vi "Router - Latency Bmk - Queue.vi"() -> ()   [LabVIEW 2016]
uses:
  <vilib>/Utility/error.llb/DialogType.ctl
  <vilib>/pximc/Initialize Writer Session (DBL).vi
  <vilib>/pximc/Initialize Reader Session (DBL).vi
  <vilib>/pximc/Connect (DBL).vi
  <vilib>/pximc/Write (DBL).vi
  <vilib>/pximc/Read (DBL).vi
  <vilib>/pximc/nipximc.lvlib
panel:
  out "Stopped?":bool=TRUE
  in  "Node 2 Reader Interface":tag="PXI1Slot2" caption="interface"
  in  "Node 2 Reader Connection ID":u16=4
  in  "Node 2 Writer Interface":tag="PXI1Slot2" caption="interface"
  in  "Node 2 Writer Connection ID":u16=3
  in  "Node 1 Reader Interface":tag="PXI1Slot2" caption="interface"
  in  "Node 1 Reader Connection ID":u16=2
  in  "Stop Button":bool
  in  "Node 1 Writer Interface":tag="PXI1Slot2" caption="interface"
  in  "Buffer Size":u64=250000 caption="buffer size"
  in  "Connection Timeout (s)":dbl=60.0 caption="timeout in seconds (-1)"
  in  "Node 1 Writer Connection ID":u16=1
  # "Node 1"
  # "Node 2"
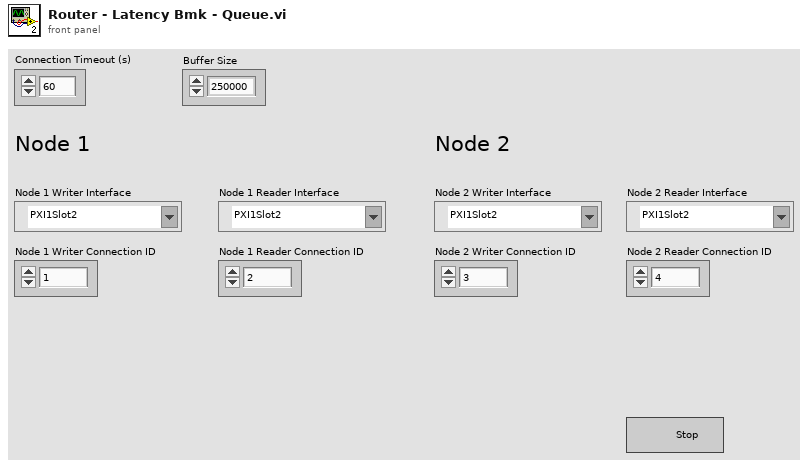
[diagram p1: front panel]
types:
  T1 = typedef "DialogType.ctl" = u16
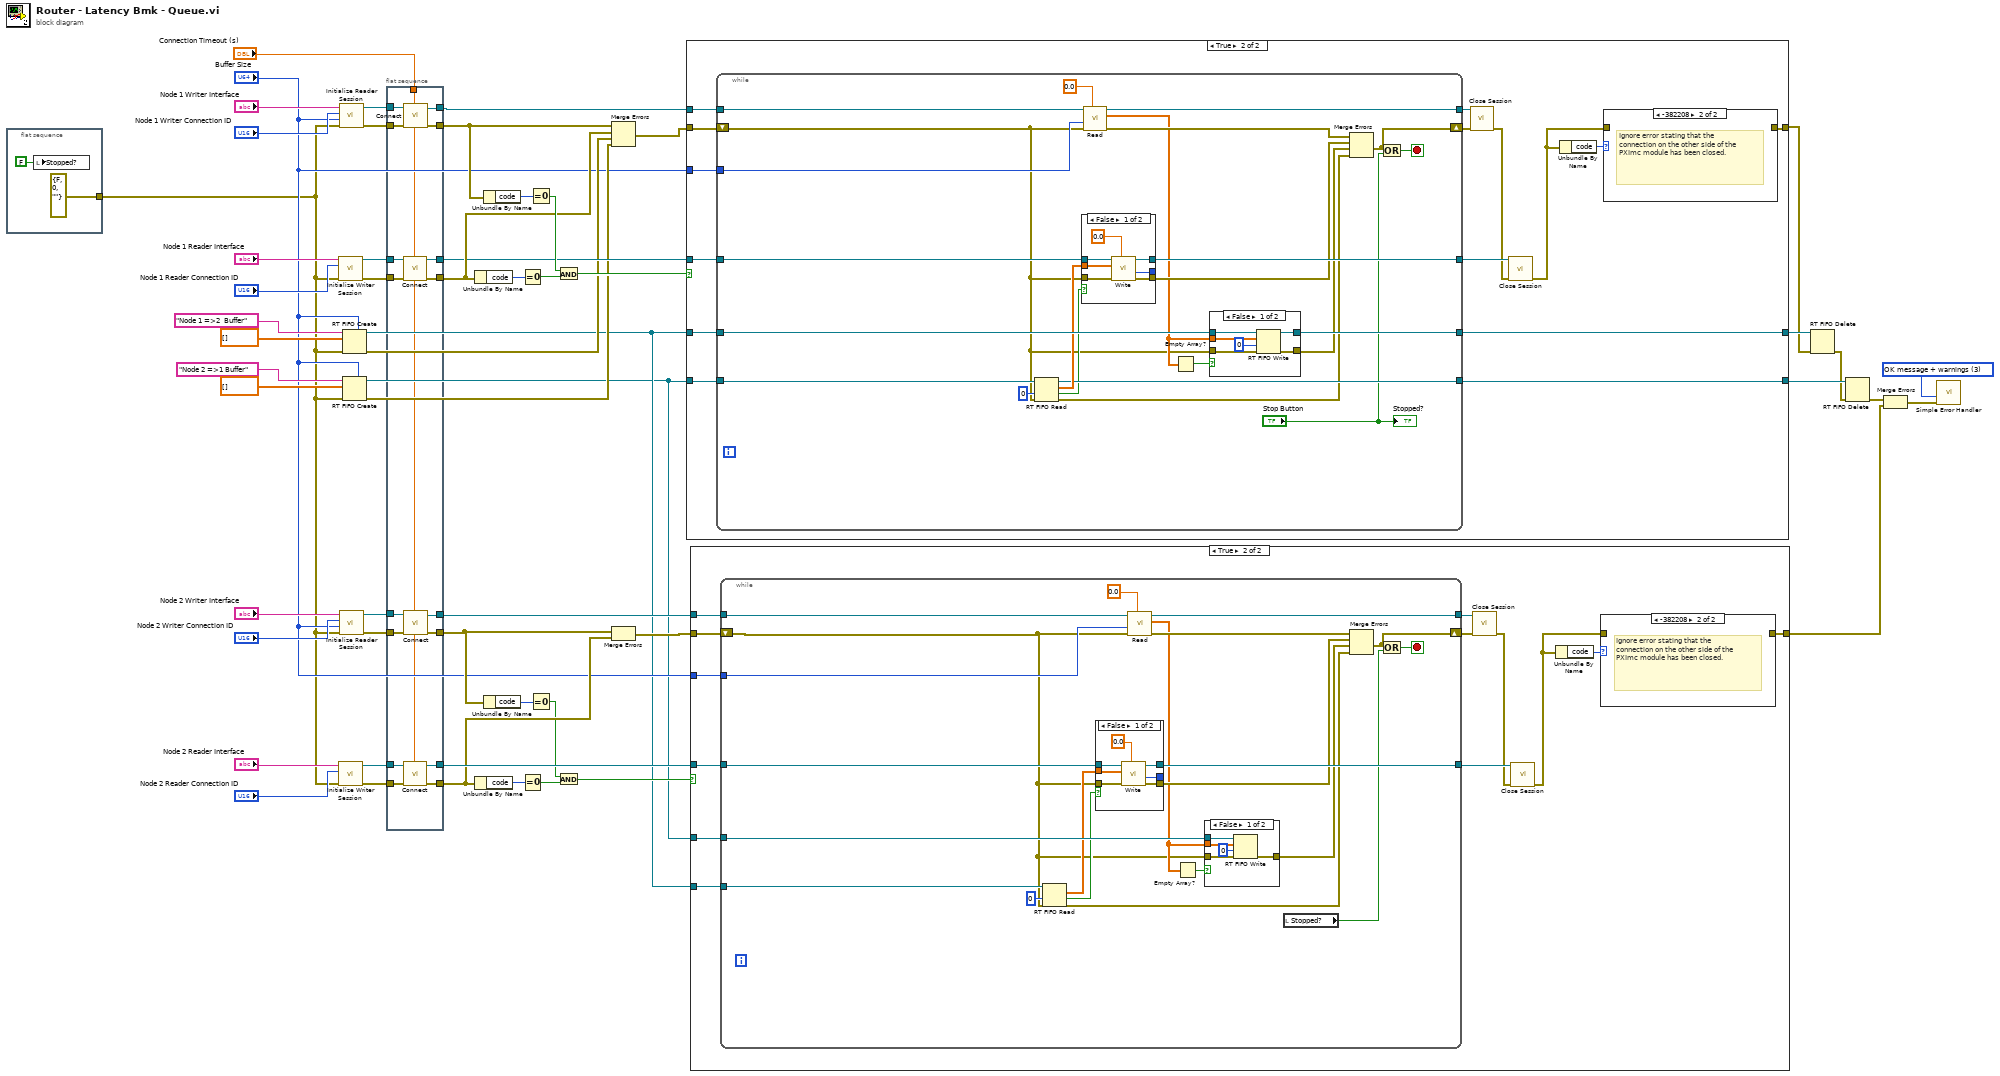
[diagram p0: block diagram]
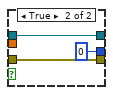
[diagram p4: hidden frame]
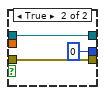
[diagram p8: hidden frame]
diagram:
  w49 = T1 3 items=["no dialog", "OK message", "continue or stop message", "OK message + warnings", "continue/stop + warnings"] ("type of dialog (OK msg:1)")
  n1 = flat-sequence {
    tunnel: [errorcluster {"status"=FALSE, "code"=0, "source"=""} ("error constant")] -> w6
    frame #0 {
      n2 = local write "Stopped?"(FALSE ("Stopped?")) -> ()
    }
  }
  n3 = call-poly <vilib>:"Initialize Writer Session.vi"("error in (no error)"=w6, "connection id (1)"="Node 1 Reader Connection ID", "interface"="Node 1 Reader Interface") -> ("error out"=w47:errorcluster, "session out"=w46:refnum<k21>)  [unwired: 7 in]
  n4 = call-poly <vilib>:"Initialize Writer Session.vi"("error in (no error)"=w6, "connection id (1)"="Node 2 Reader Connection ID", "interface"="Node 2 Reader Interface") -> ("error out"=w15:errorcluster, "session out"=w16:refnum<k21>)  [unwired: 7 in]
  n5 = call-poly <vilib>:"Initialize Reader Session.vi"("error in (no error)"=w6, "buffer size"="Buffer Size", "writer's connection id (1)"="Node 1 Writer Connection ID", "interface"="Node 1 Writer Interface") -> ("error out"=w53:errorcluster, "session out"=w54:refnum<k21>)  [unwired: 6 in]
  n6 = call-poly <vilib>:"Initialize Reader Session.vi"("error in (no error)"=w6, "buffer size"="Buffer Size", "writer's connection id (1)"="Node 2 Writer Connection ID", "interface"="Node 2 Writer Interface") -> ("error out"=w10:errorcluster, "session out"=w9:refnum<k21>)  [unwired: 6 in]
  n7 = RT FIFO Create(0:"Node 1 =>2  Buffer" ("name (unnamed)"), 1:dbl[] [] ("data"), 3:w6, 6:"Buffer Size") -> (8:w5:refnum<k33>, 11:w26:errorcluster)  [unwired: 4 in, 1 out]
  n8 = RT FIFO Create(0:"Node 2 =>1 Buffer" ("name (unnamed)"), 1:dbl[] [] ("data"), 3:w6, 6:"Buffer Size") -> (8:w4:refnum<k33>, 11:w33:errorcluster)  [unwired: 4 in, 1 out]
  n9 = flat-sequence {
    tunnel: w54 -> [w74]
    tunnel: w53 -> [w73]
    tunnel: [w72] -> w52
    tunnel: w47 -> [w71]
    tunnel: w46 -> [w70]
    tunnel: [w69] -> w39
    tunnel: [w68] -> w38
    tunnel: "Connection Timeout (s)" -> [w58]
    tunnel: [w67] -> w35
    tunnel: [w66] -> w25
    tunnel: [w65] -> w24
    tunnel: [w64] -> w23
    tunnel: w16 -> [w63]
    tunnel: w15 -> [w62]
    tunnel: [w61] -> w11
    tunnel: w10 -> [w60]
    tunnel: w9 -> [w59]
    frame #0 {
      n10 = call-poly <vilib>:"Connect.vi"("timeout in seconds (-1)"=w58, "error in (no error)"=w71, "session in"=w70) -> ("error out"=w68:errorcluster, "session out"=w67:refnum<k21>)  [unwired: 7 in]
      n11 = call-poly <vilib>:"Connect.vi"("timeout in seconds (-1)"=w58, "error in (no error)"=w62, "session in"=w63) -> ("error out"=w65:errorcluster, "session out"=w66:refnum<k21>)  [unwired: 7 in]
      n12 = call-poly <vilib>:"Connect.vi"("timeout in seconds (-1)"=w58, "error in (no error)"=w73, "session in"=w74) -> ("error out"=w69:errorcluster, "session out"=w72:refnum<k21>)  [unwired: 7 in]
      n13 = call-poly <vilib>:"Connect.vi"("timeout in seconds (-1)"=w58, "error in (no error)"=w60, "session in"=w59) -> ("error out"=w64:errorcluster, "session out"=w61:refnum<k21>)  [unwired: 7 in]
    }
  }
  n14 = Unbundle By Name(w38) -> ("code"=w44:i32)
  n15 = Unbundle By Name(w24) -> ("code"=w18:i32)
  n16 = Unbundle By Name(w39) -> ("code"=w50:i32)
  n17 = Unbundle By Name(w23) -> ("code"=w13:i32)
  n18 = Equal To 0?(x=w44) -> (x = 0?=w41:bool)
  n19 = Equal To 0?(x=w18) -> (x = 0?=w21:bool)
  n20 = Equal To 0?(x=w50) -> (x = 0?=w42:bool)
  n21 = Equal To 0?(x=w13) -> (x = 0?=w20:bool)
  n22 = And(x=w42, y=w41) -> (x .and. y?=w43:bool)
  n23 = And(x=w20, y=w21) -> (x .and. y?=w19:bool)
  n24 = Merge Errors(w39, w38, w26, w33) -> (w40:errorcluster)
  n25 = Merge Errors(w23, w24) -> (w22:errorcluster)
  n26 = case shown="True" w43 {
    tunnel: w40 -> [w77 w92]
    tunnel: w52 -> [_ w91]
    tunnel: [w77 w89] -> w28
    tunnel: w5 -> [w76 w86]
    tunnel: "Buffer Size" -> [_ w85]
    tunnel: w35 -> [_ w84]
    tunnel: w4 -> [w75 w83]
    tunnel: [w76 w82] -> w30
    tunnel: [w75 w80] -> w29
    frame False {
      # "The connection was not successful for some reason."
    }
    frame True {
      n27 = while {
        tunnel: w91 -> [w115]
        tunnel: [w114] -> w90
        shift-right: [w100] -> w87
        shift-left: w92 -> [w93]
        tunnel: w86 -> [w113]
        tunnel: w85 -> [w112]
        tunnel: w84 -> [w111]
        tunnel: w83 -> [w110]
        tunnel: [w108] -> w82
        tunnel: [w107] -> w80
        tunnel: [w106] -> w81
        stop <- w101 stop-if-true
        n28 = RT FIFO Read(0:w110, 2:0 ("timeout in ms (0)"), 3:w93) -> (8:w107:refnum<k33>, 9:w109:dbl[], 10:w96:bool, 11:w102:errorcluster)  [unwired: 1 in, 1 out]
        n29 = case shown="False" w96 {
          tunnel: w111 -> [w130 w133]
          tunnel: w109 -> [w129 _]
          tunnel: w93 -> [w128 w131]
          tunnel: [w127 u32 0 ("number of elements written")] -> _
          tunnel: [w126 w133] -> w106
          tunnel: [w125 w131] -> w104
          frame False {
            n30 = call-poly <vilib>:"Write.vi"("timeout in seconds (5)"=0.0, "error in (no error)"=w128, "data"=w129, "session in"=w130) -> ("error out"=w125:errorcluster, "number of elements written"=w127:u32, "session out"=w126:refnum<k21>)  [unwired: 5 in]
          }
          frame True {
          }
        }
        n31 = call-poly <vilib>:"Read.vi"("timeout in seconds (5)"=0.0, "error in (no error)"=w93, "number of elements"=w112, "session in"=w115) -> ("error out"=w105:errorcluster, "data"=w95:dbl[], "session out"=w114:refnum<k21>)  [unwired: 5 in]
        n32 = Empty Array?(array=w95) -> (empty?=w94:bool)
        n33 = case shown="False" w94 {
          tunnel: w95 -> [w121 _]
          tunnel: w113 -> [w120 w123]
          tunnel: w93 -> [w119 w122]
          tunnel: [w118 w123] -> w108
          tunnel: [w117 w122] -> w103
          frame False {
            n34 = RT FIFO Write(0:w120, 1:w121, 2:0 ("timeout in ms (0)"), 3:w119) -> (8:w118:refnum<k33>, 11:w117:errorcluster)  [unwired: 1 in, 2 out]
          }
          frame True {
          }
        }
        n35 = Merge Errors(w105, w104, w103, w102) -> (w100:errorcluster)
        n36 = Or(x=w100, y="Stop Button") -> (x .or. y?=w101:bool)
        "Stopped?" <- "Stop Button"
      }
      n37 = call <vilib>:"Close Session.vi"("error in (no error)"=w87, "session in"=w90) -> ("error out"=w79:errorcluster)  [unwired: 9 in]
      n38 = call <vilib>:"Close Session.vi"("error in (no error)"=w79, "session in"=w81) -> ("error out"=w78:errorcluster)  [unwired: 9 in]
      n39 = Unbundle By Name(w78) -> ("code"=w88:i32)
      n40 = case shown="-382208" w88 {
        tunnel: w78 -> [w134 _]
        tunnel: [w134 _] -> w89
        frame 0, Default {
        }
        frame -382208 {
          # "Ignore error stating that the connection on the other side of the PXImc module has been closed."
        }
      }
    }
  }
  n41 = case shown="True" w19 {
    tunnel: w22 -> [w135 w148]
    tunnel: w11 -> [_ w147]
    tunnel: [w135 w145] -> w2
    tunnel: w4 -> [_ w142]
    tunnel: "Buffer Size" -> [_ w141]
    tunnel: w25 -> [_ w140]
    tunnel: w5 -> [_ w139]
    frame False {
      # "The connection was not successful for some reason."
    }
    frame True {
      n42 = while {
        tunnel: w147 -> [w169]
        tunnel: [w168] -> w146
        shift-right: [w156] -> w143
        shift-left: w148 -> [w149]
        tunnel: w142 -> [w167]
        tunnel: w141 -> [w166]
        tunnel: w140 -> [w165]
        tunnel: w139 -> [w164]
        tunnel: [w162] -> w138
        stop <- w157 stop-if-true
        n43 = RT FIFO Read(0:w164, 2:0 ("timeout in ms (0)"), 3:w149) -> (9:w163:dbl[], 10:w152:bool, 11:w158:errorcluster)  [unwired: 1 in, 2 out]
        n44 = case shown="False" w152 {
          tunnel: w165 -> [w182 w184]
          tunnel: w163 -> [w181 _]
          tunnel: w149 -> [w180 w185]
          tunnel: [w179 u32 0 ("number of elements written")] -> _
          tunnel: [w178 w184] -> w162
          tunnel: [w177 w185] -> w160
          frame False {
            n45 = call-poly <vilib>:"Write.vi"("timeout in seconds (5)"=0.0, "error in (no error)"=w180, "data"=w181, "session in"=w182) -> ("error out"=w177:errorcluster, "number of elements written"=w179:u32, "session out"=w178:refnum<k21>)  [unwired: 5 in]
          }
          frame True {
          }
        }
        n46 = call-poly <vilib>:"Read.vi"("timeout in seconds (5)"=0.0, "error in (no error)"=w149, "number of elements"=w166, "session in"=w169) -> ("error out"=w161:errorcluster, "data"=w151:dbl[], "session out"=w168:refnum<k21>)  [unwired: 5 in]
        n47 = Empty Array?(array=w151) -> (empty?=w150:bool)
        n48 = case shown="False" w150 {
          tunnel: w151 -> [w174 _]
          tunnel: w167 -> [w173 _]
          tunnel: w149 -> [w172 w175]
          tunnel: [w171 w175] -> w159
          frame False {
            n49 = RT FIFO Write(0:w173, 1:w174, 2:0 ("timeout in ms (0)"), 3:w172) -> (11:w171:errorcluster)  [unwired: 1 in, 3 out]
          }
          frame True {
          }
        }
        n50 = local read "Stopped?"() -> (w155:bool)
        n51 = Merge Errors(w161, w160, w159, w158) -> (w156:errorcluster)
        n52 = Or(x=w156, y=w155) -> (x .or. y?=w157:bool)
      }
      n53 = call <vilib>:"Close Session.vi"("error in (no error)"=w143, "session in"=w146) -> ("error out"=w137:errorcluster)  [unwired: 9 in]
      n54 = call <vilib>:"Close Session.vi"("error in (no error)"=w137, "session in"=w138) -> ("error out"=w136:errorcluster)  [unwired: 9 in]
      n55 = Unbundle By Name(w136) -> ("code"=w144:i32)
      n56 = case shown="-382208" w144 {
        tunnel: w136 -> [w186 _]
        tunnel: [w186 _] -> w145
        frame 0, Default {
        }
        frame -382208 {
          # "Ignore error stating that the connection on the other side of the PXImc module has been closed."
        }
      }
    }
  }
  n57 = RT FIFO Delete(0:w30, 3:w28) -> (11:w27:errorcluster)  [unwired: 1 in]
  n58 = RT FIFO Delete(0:w29, 3:w27) -> (11:w3:errorcluster)  [unwired: 1 in]
  n59 = Merge Errors(w3, w2) -> (w1:errorcluster)
  n60 = call <vilib>:"Simple Error Handler.vi"("type of dialog (OK msg:1)"=w49, "error in (no error)"=w1) -> ()  [unwired: 3 in, 5 out]
